vi "test_libssh2_sftp_shutdown.vi"() -> ()   [LabVIEW 2017, in "integration_tests.lvlib"]
uses:
  integration_tests.lvlib
  support/support.lvlib
  libssh2/libssh2.lvlib
  <vilib>/PNR/Transparent Assertions/Transparent Assertions/Transparent Assertions.lvlib
panel:
  out "error out":errorcluster
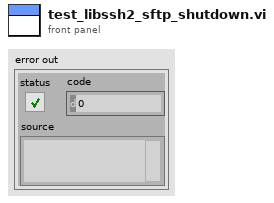
[diagram p1: front panel]
types:
  T1 = typedef "libssh2.lvlib/Session Refnum.ctl" = refnum<k1>
  T2 = typedef "libssh2.lvlib/SFTP Refnum.ctl" = refnum<k1>
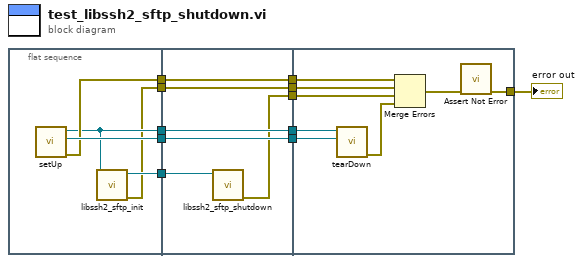
[diagram p0: block diagram]
diagram:
  n1 = flat-sequence {
    tunnel: [w13] -> w11
    tunnel: [w16] -> w10
    tunnel: [w15] -> w6
    tunnel: [w14] -> w5
    tunnel: [w12] -> w4
    tunnel: w11 -> [w22]
    tunnel: w10 -> [w21]
    tunnel: [w22] -> w9
    tunnel: [w21] -> w8
    tunnel: [w20] -> w7
    tunnel: w6 -> [w20]
    tunnel: w5 -> [w19]
    tunnel: w4 -> [w18]
    tunnel: [w18] -> w3
    tunnel: [w17] -> w1
    tunnel: w9 -> [w30]
    tunnel: w8 -> [w29]
    tunnel: w7 -> [w28]
    tunnel: w3 -> [w26]
    tunnel: [w24] -> w2
    tunnel: w1 -> [w23]
    frame #0 {
      n2 = call "setUp.vi"() -> ("error out"=w15:errorcluster, "connection ID"=w16:refnum<k5>, "session"=w13:T1)  [unwired: 9 in]
      n3 = call "libssh2_sftp_init.vi"("session"=w13) -> ("error out"=w12:errorcluster, "sftp"=w14:T2)  [unwired: 9 in]
    }
    frame #1 {
      n4 = call "libssh2_sftp_shutdown.vi"("sftp"=w19) -> ("error out"=w17:errorcluster)  [unwired: 10 in]
    }
    frame #2 {
      n5 = call "tearDown.vi"("connection ID"=w29, "session"=w30) -> ("error out"=w27:errorcluster)  [unwired: 9 in]
      n6 = Merge Errors(w28, w26, w23, w27) -> (w25:errorcluster)
      n7 = call <vilib>:"Assert Not Error.vi"("error in (no error)"=w25) -> ("error out"=w24:errorcluster)  [unwired: 10 in]
    }
  }
  "error out" <- w2
